vi "Init Control.vi"(5 "Group":refnum<class "Group.lvclass">, 6 "Period ms":i64, 7 "VolatusAPI":refnum<class "VolatusAPI.lvclass">, 8 "error in (no error)":errorcluster, 9 "Control MsgQ":refnum<class "MessageQ.lvclass">, 10 "Config Element":refnum<class "Config Element.lvclass">, 11 "Valve in":refnum<class "PeriodicControl.lvclass">) -> (0 "error out":errorcluster, 3 "Valve out":refnum<class "PeriodicControl.lvclass">)   [LabVIEW 2020, in "VolatusControl.lvlib" / "PeriodicControl.lvclass"]
uses:
  PeriodicControl.lvclass
  lv-cdm/CDM-Config/Config Element/Config Element.lvclass
  Volatus/VolatusAPI/VolatusAPI.lvclass
  Volatus/MessageQ/MessageQ.lvclass
  lv-vecto/Vecto/Group/Group.lvclass
  C:/dev/lv20CE/relink/lv-vecto/Vecto/GroupAbstract/GroupAbstract.lvclass
  Volatus/Module Identity/Module Identity.lvclass/Module Identity.ctl
  PeriodicControl.lvclass/PeriodicControl.ctl
  Volatus/Module Identity/Create.vi
  Volatus/Module Identity/Module Identity.lvclass
  C:/dev/lv20CE/relink/lv-volatus/Volatus/Identity/Identity.lvclass
  lv-cdm/CDM-Config/Config Element/Owner.vi
  lv-cdm/CDM-Config/Config Manager/Lookup Descendant.vi
  Volatus/VolatusAPI/Lookup Channel Info.vi
  Volatus/VolatusAPI/Lookup Q.vi
  lv-cdm/CDM-Config/Config Filter/Config Lookup.lvclass
  lv-vecto/Vecto/GroupAbstract/GroupAbstract.lvclass
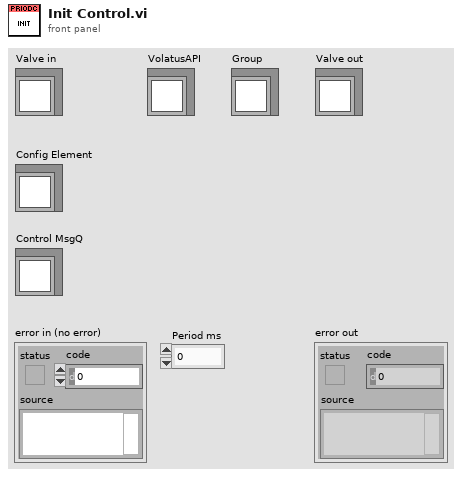
[diagram p1: front panel]
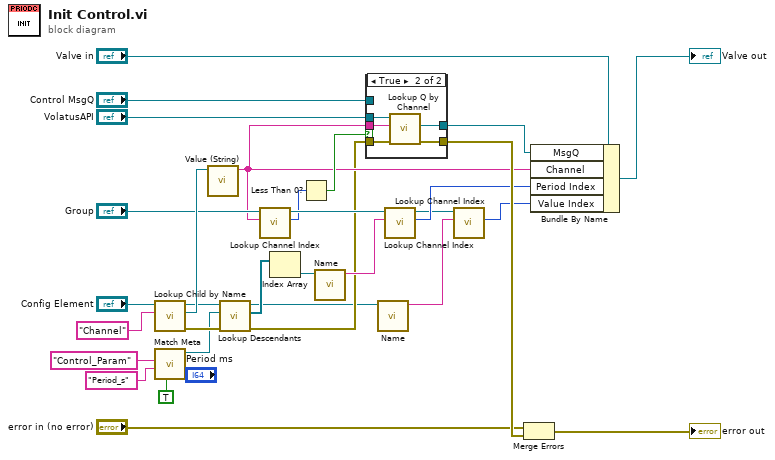
[diagram p0: block diagram]
diagram:
  n1 = call "Lookup Child by Name.vi"("Name"="Channel", "Config Element in"="Config Element") -> ("error out"=w21:errorcluster, "Child"=w26:refnum<class "Config Element.lvclass">, "Config Element out"=w22:refnum<class "Config Element.lvclass">)  [unwired: 6 in, 1 out]
  n2 = call "Match Meta.vi"("Exact Value (F)"=TRUE, "Value (Any)"="Period_s" ("Name"), "Name"="Control_Param") -> ("Config Lookup out"=w20:refnum<class "Config Lookup.lvclass">)  [unwired: 7 in, 1 out]
  n3 = call "Value (String).vi"("Config Element in"=w26) -> ("String Value"=w10:string)  [unwired: 9 in, 1 out]
  n4 = call "Lookup Descendants.vi"("error in (no error)"=w21, "Lookup"=w20, "Config Element in"=w22) -> ("error out"=w6:errorcluster, "Descendants"=w19:refnum<class "Config Element.lvclass">[], "Config Element out"=w4:refnum<class "Config Element.lvclass">)  [unwired: 6 in]
  n5 = call "Lookup Channel Index.vi"("Channel Name"=w10, "GroupAbstract in"="Group") -> ("Index"=w13:i32, "GroupAbstract out"=w14:refnum<class "Group.lvclass">)  [unwired: 7 in, 1 out]
  n6 = Index Array(array=w19) -> (element=w18:refnum<class "Config Element.lvclass">)  [unwired: 1 in]
  n7 = Less Than 0?(x=w13) -> (x < 0?=w11:bool)
  n8 = call "Name.vi"("Config Element in"=w18) -> ("Name"=w17:string)  [unwired: 9 in, 1 out]
  n9 = case shown="True" w11 {
    tunnel: "VolatusAPI" -> [_ w38]
    tunnel: w10 -> [_ w37]
    tunnel: [w33 w36] -> w9
    tunnel: "Control MsgQ" -> [w33 _]
    tunnel: w6 -> [w32 w35]
    tunnel: [w32 w34] -> w31
    frame False {
    }
    frame True {
      n10 = call "Lookup Q by Channel.vi"("error in (no error)"=w35, "Channel Name"=w37, "VolatusAPI in"=w38) -> ("error out"=w34:errorcluster, "MessageQ"=w36:refnum<class "MessageQ.lvclass">)  [unwired: 6 in, 1 out]
    }
  }
  n11 = call "Name.vi"("Config Element in"=w4) -> ("Name"=w2:string)  [unwired: 9 in, 1 out]
  n12 = call "Lookup Channel Index.vi"("Channel Name"=w17, "GroupAbstract in"=w14) -> ("Index"=w7:i32, "GroupAbstract out"=w3:refnum<class "Group.lvclass">)  [unwired: 7 in, 1 out]
  n13 = call "Lookup Channel Index.vi"("Channel Name"=w2, "GroupAbstract in"=w3) -> ("Index"=w1:i32)  [unwired: 7 in, 2 out]
  n14 = Merge Errors("error in (no error)", w31) -> (→"error out":errorcluster)
  n15 = Bundle By Name(cluster="Valve in", "MsgQ"=w9, "Channel"=w10, "Period Index"=w7, "Value Index"=w1) -> (→"Valve out":refnum<class "PeriodicControl.lvclass">)
